vi "Task Manager.vi"() -> ()   [LabVIEW 2019, in "Task Manager.lvlib"]
doc: "This template is for the Queued Message Handler design pattern.\n\nThe Event Handling Loop generates messages based on user interface actions.\n\nThe Message Handling Loop processes messages generated by the Event Handling Loop, or by other messages. The messages are string values, so new messages can be added easily to the Message Cases case structure in the Message Handling Loop. Each message cluster can also provide an optional value for Message Data, which is a variant that can be converted to whatever message-specific data is required.a"
uses:
  Task Manager.lvlib
  Shared/TypeDefs/Queue Info.ctl
  Data.ctl
  Message Queue/State Name.ctl
  <vilib>/event_ctls.llb/usereventprio.ctl
  0c61461a-fa07-4497-8c8c-8d3ef654e9c8.vi
  bad579f2-958a-4e04-a1a5-1778729f7708.vi
  681f6a39-68c9-4eb8-ab39-fd2fc03f9966.vi
  <vilib>/Utility/error.llb/Clear Errors.vi
  Message Queue/Enqueue (Single).vi
  <vilib>/Utility/error.llb/Error Cluster From Error Code.vi
  Message Queue/Enqueue (Array).vi
  Message Queue/Reference Queue.vi
  Message Queue/Message Queue.lvlib
panel:
  in  "States Calling Info":cluster{"Queue Info":T1, "Show FP":bool}[](array[cluster])=[{"Queue Info"={"Module"="Asfand.lvlib", "State Name"="Initialize Data", "State Dequeue Time"="11 : 57 : 24.167319 AM", "Interval"="505.162129331m", "Call Chain"="Zeshan.lvlib:Zeshan.vi --> Message Queue.lvlib:Global Message Queue.vi", "# elements in queue"=0}, "Show FP"=FALSE}, {"Queue Info"={"Module"="Hamza.lvlib", "State Name"="[Event Structure] Update Data", "State Dequeue Time"="11 : 57 : 24.030312 AM", "Interval"="505.018426931m", "Call Chain"="Hamza.lvlib:Hamza.vi", "# elements in queue"=0}, "Show FP"=FALSE}, {"Queue Info"={"Module"="Zeshan.lvlib", "State Name"="[Event Structure] Update Data", "State Dequeue Time"="11 : 57 : 24.090315 AM", "Interval"="801.170772896m", "Call Chain"="Zeshan.lvlib:Zeshan.vi", "# elements in queue"=0}, "Show FP"=FALSE}]
  out "Modules Names":string[](array[string])=["Asfand", "Hamza", "Zeshan", "Acquire Mouse", "Task Manager"]
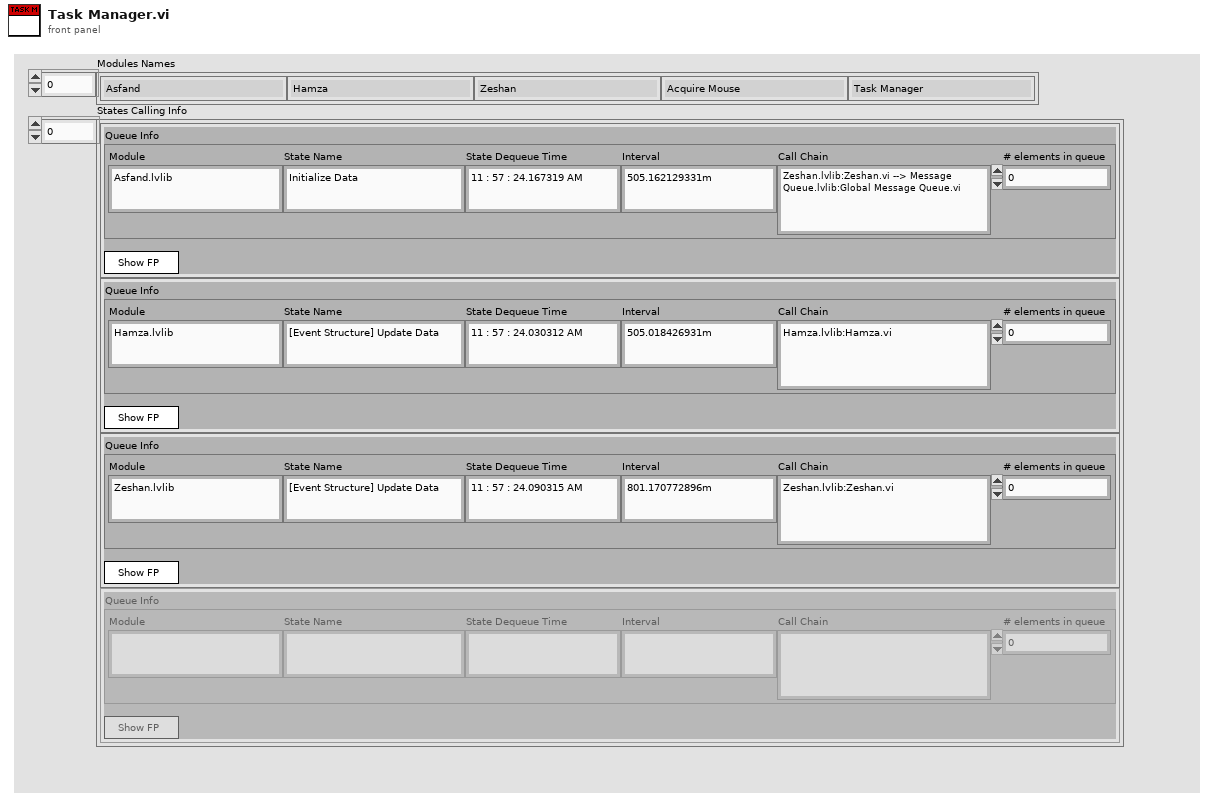
[diagram p1: front panel]
types:
  T1 = typedef "Queue Info.ctl" = cluster{"Module":string, "State Name":string, "State Dequeue Time":string, "Interval":string, "Call Chain":string, "# elements in queue":i32}
  T2 = typedef "Task Manager.lvlib/State Name.ctl" = enum16{"Default", "Initialize", "Re-Initialize", "Initialize Data", "Initialize Panel", "[Event Structure] Update Data", "Get Modules", "Add State Info Clone", "Get Queue Sizes", "Get States Calling Info", "Error", "Exit"}
  T3 = typedef "Task Manager.lvlib/Data.ctl" = cluster{"Exit":bool, "States":T2, "Refs":cluster{"Modules":refnum<vi>[], "FGVs":refnum<vi>[]}, "Modules":string[], "Queues Status":cluster{"max queue size":i32, "queue name":string, "# pending remove":i32, "# pending insert":i32, "# elements in queue":i32, "elements":cluster{"Custom State Name":string, "Defined State Name":variant, "Call Chain":string[], "Message Data":variant}[]}[], "States Calling Info":cluster{"Queue Info":T1, "Show FP":bool}[]}
  T4 = typedef "Message Queue Ref.ctl" = refnum<queue>
  T5 = typedef "Message Queue.lvlib/State Name.ctl" = enum16{"Default", "Initialize", "Initialize Data", "Initialize Modules", "Initialize Panel", "Close FP", "Open FP", "Initialize Menu", "Mode", "Update Subpanel", "Error", "Open Help", "About", "Open WebResources", "Exit"}
  T6 = typedef "usereventprio.ctl" = enum32{"high priority", "normal priority"}
  T7 = cluster{"max queue size":i32, "queue name":string, "# pending remove":i32, "# pending insert":i32, "# elements in queue":i32, "elements":cluster{"Custom State Name":string, "Defined State Name":variant, "Call Chain":string[], "Message Data":variant}[]}
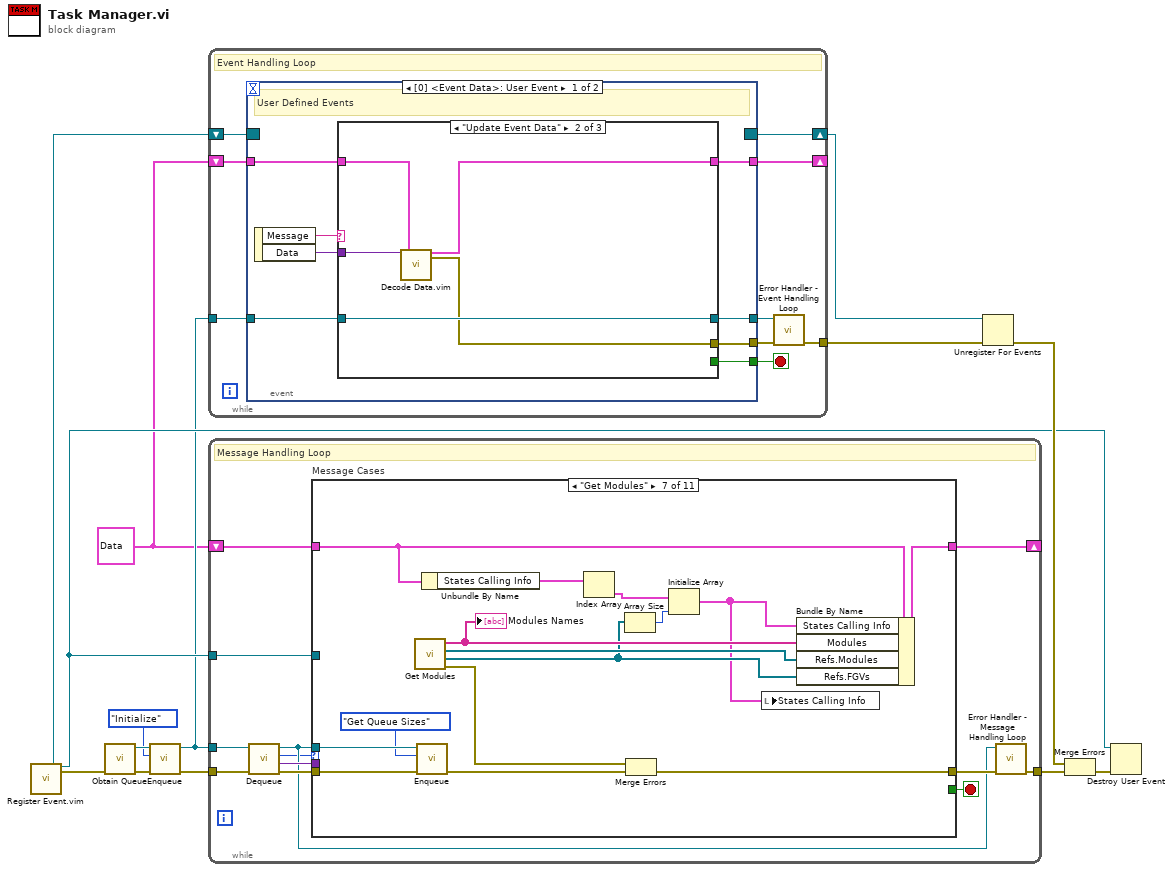
[diagram p0: block diagram]
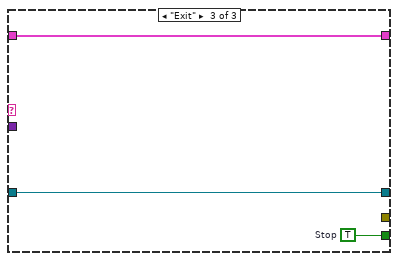
[diagram p3: hidden frame]
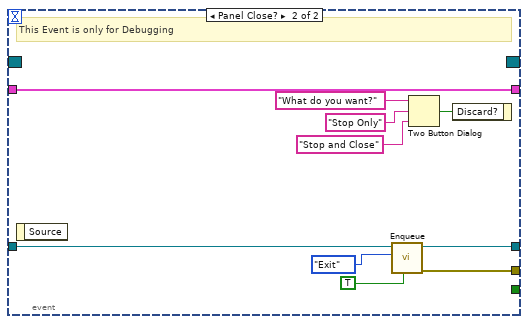
[diagram p4: hidden frame]
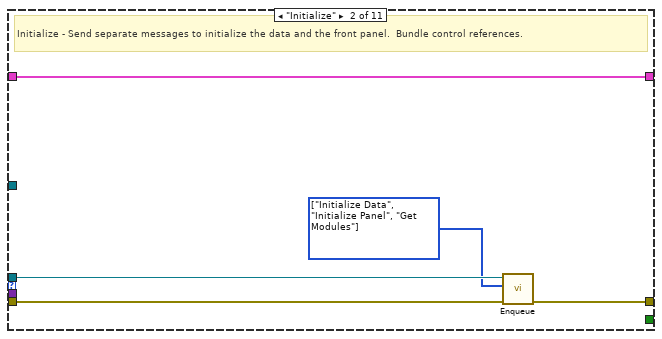
[diagram p6: hidden frame]
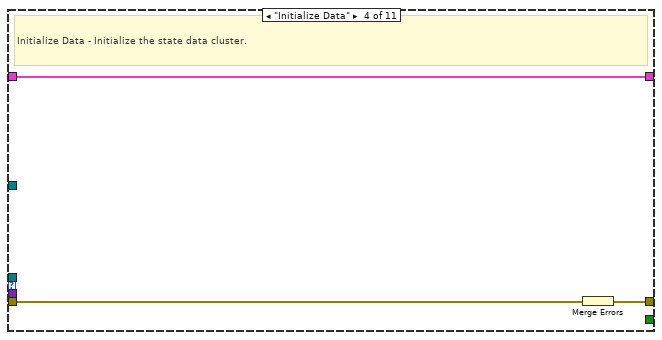
[diagram p8: hidden frame]
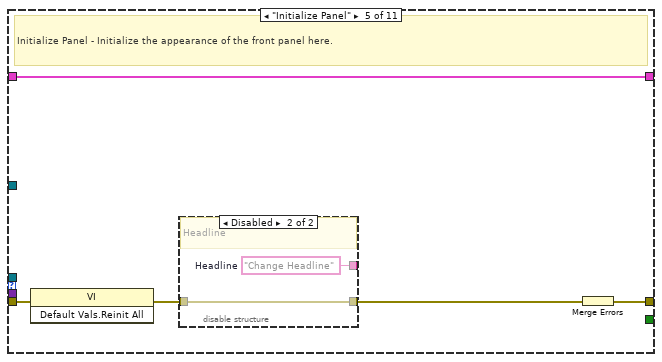
[diagram p9: hidden frame]
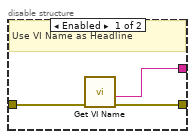
[diagram p10: hidden frame]
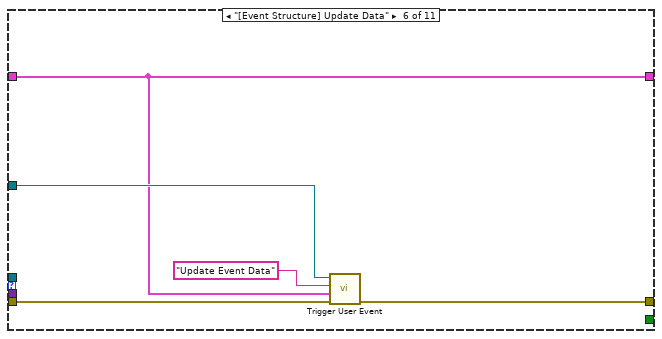
[diagram p11: hidden frame]
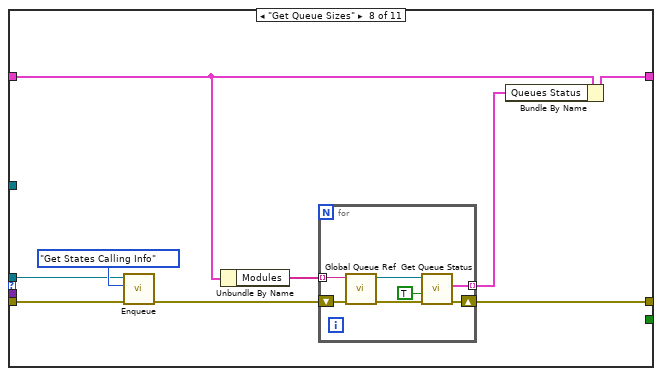
[diagram p12: hidden frame]
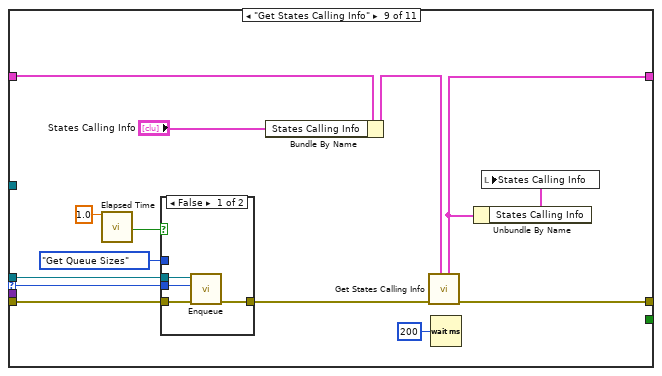
[diagram p13: hidden frame]
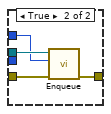
[diagram p14: hidden frame]
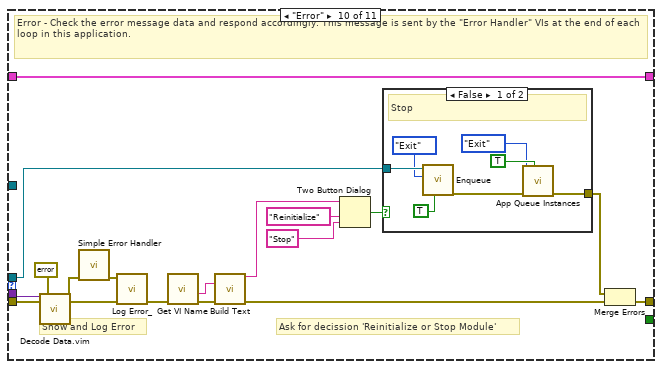
[diagram p15: hidden frame]
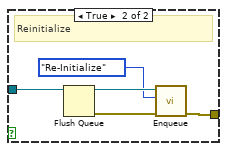
[diagram p16: hidden frame]
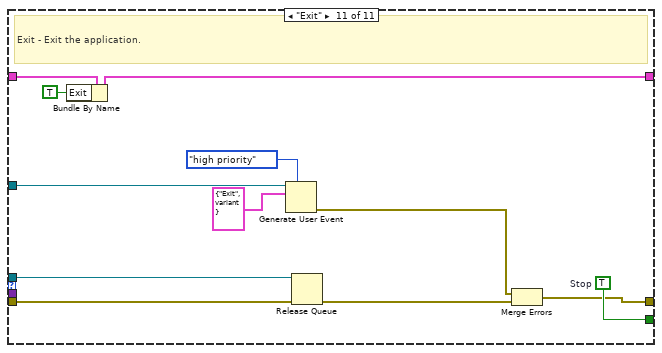
[diagram p17: hidden frame]
diagram:
  w3 = T3 {"Exit"=FALSE, "States"=enum."Initialize", "Refs"={"Modules"=[], "FGVs"=[]}, "Modules"=[], "Queues Status"=[], "States Calling Info"=[]} ("Data")
  n1 = call "Register Event.vim"() -> ("Registration"=w2:refnum<event-registration>, "user event out"=w5:refnum<user-event>, "error out"=w6:errorcluster)  [unwired: 17 in]
  n2 = call "Obtain Queue.vi"("error in (no error)"=w6) -> ("error out"=w10:errorcluster, "Message out"=w11:T4)  [unwired: 9 in]
  n3 = call-poly "Enqueue.vi"("error in (no error)"=w10, "States"=State_Name."Initialize", "Message Queue"=w11) -> ("error out"=w9:errorcluster, "Message Queue dub"=w4:T4)  [unwired: 7 in]
  n4 = while {
    tunnel: w4 -> [w23]
    shift-right: [w15] -> w8
    shift-left: w2 -> [w16]
    tunnel: [w20] -> w12
    shift-right: [w17] -> _
    shift-left: w3 -> [w18]
    stop <- w22 stop-if-true
    # "Event Handling Loop"
    n5 = event shown="[0] <Event Data>: User Event" {
      selector: w16 -> [_ _]
      dyn-events: [_ _] -> w15
      timeout: _ -> [_ _]
      tunnel: [w31 _] -> w22
      tunnel: w23 -> [w28 w44]
      tunnel: [w30 w45] -> w19
      tunnel: [w29 w46] -> w21
      tunnel: w18 -> [w26 w42]
      tunnel: [w27 w42] -> w17
      event User Event {
        # "User Defined Events"
        n6 = event-data() -> ("Message"=w25:string, "Data"=w24:variant)  [unwired: 1 in]
        n7 = case shown="\"Update Event Data\"" w25 {
          tunnel: [_ _ w41] -> w31
          tunnel: [_ w34 _] -> w30
          tunnel: w24 -> [_ w38 _]
          tunnel: [w33 w35 w40] -> w29
          tunnel: w28 -> [w33 w35 w40]
          tunnel: [w32 w36 w39] -> w27
          tunnel: w26 -> [w32 w37 w39]
          frame Default {
          }
          frame "Update Event Data" {
            n8 = call "Decode Data.vim"("Data"=w38, "Type/Default value"=w37) -> ("Data out"=w36:T3, "error out"=w34:errorcluster)  [unwired: 16 in]
          }
          frame "Exit" {
            w41 = TRUE  # Stop
          }
        }
      }
      event Panel Close? {
        # "This Event is only for Debugging"
        n9 = event-data() -> ()  [unwired: 1 in, 1 out]
        n10 = call-poly "Enqueue.vi"("Priority Message? Array"=TRUE ("Priority Message? (F)"), "States"=State_Name."Exit" ("Array"), "Message Queue"=w44) -> ("error out"=w45:errorcluster, "Message Queue dub"=w46:T4)  [unwired: 7 in]
        n11 = Two Button Dialog(message="What do you want?", 1:"Stop and Close" ("F button name (\"Cancel\")"), 2:"Stop Only" ("T button name (\"OK\")")) -> (T button?=w48:bool)
        n12 = event-data("Discard?"=w48) -> ()  [unwired: 1 in, 1 out]
      }
    }
    n13 = call "Error Handler - Event Handling Loop.vi"("error in (no error)"=w19, "Message Queue"=w21) -> ("dup error in"=w20:errorcluster)  [unwired: 8 in, 1 out]
  }
  n14 = while {
    tunnel: w4 -> [w58]
    tunnel: w9 -> [w61]
    tunnel: [w57] -> w14
    shift-right: [w53] -> _
    shift-left: w3 -> [w63]
    tunnel: w5 -> [w52]
    stop <- w62 stop-if-true
    # "Message Handling Loop"
    n15 = call "Dequeue.vi"("error in (no error)"=w61, "Message Queue"=w58) -> ("error out"=w60:errorcluster, "Message Data"=w59:variant, "State"=w54:T2, "Message Queue dub"=w55:T4)  [unwired: 4 in, 2 out]
    n16 = case "Message Cases" shown="\"Get Modules\"" w54 {
      selector: w54 -> [_ _ _ _ _ _ _ _ w128 _ _]
      tunnel: w55 -> [_ w68 _ _ _ _ w99 w106 w127 w150 w185]
      tunnel: w60 -> [w65 w69 w72 w73 w78 w90 w101 w109 w126 w148 w181]
      tunnel: [w65 w70 w72 w75 w80 w89 w103 w114 w135 w149 w182] -> w56
      tunnel: w63 -> [w64 w67 w71 w74 w79 w87 w97 w112 w134 w161 w179]
      tunnel: [_ _ _ _ _ _ _ _ _ _ w184] -> w62
      tunnel: w59 -> [_ _ _ _ _ _ _ _ _ w145 _]
      tunnel: [w64 w67 w71 w74 w79 w87 w105 w111 w133 w161 w175] -> w53
      tunnel: w52 -> [_ _ _ _ _ w88 _ _ _ _ w180]
      frame "Default", Default {
      }
      frame "Initialize" {
        w66 = T2[] [enum."Initialize Data", enum."Initialize Panel", enum."Get Modules"] items=["Default", "Initialize", "Re-Initialize", "Initialize Data", "Initialize Panel", "[Event Structure] Update Data", "Get Modules", "Add State Info Clone", "Get Queue Sizes", "Get States Calling Info", "Error", "Exit"] ("Array")
        # "Initialize - Send separate messages to initialize the data and the front panel.  Bundle control references."
        n17 = call-poly "Enqueue.vi"("error in (no error)"=w69, "States"=w66, "Message Queue"=w68) -> ("error out"=w70:errorcluster)  [unwired: 7 in, 1 out]
      }
      frame "Re-Initialize" {
      }
      frame "Initialize Data" {
        # "Initialize Data - Initialize the state data cluster."
        n18 = Merge Errors(w73) -> (w75:errorcluster)
      }
      frame "Initialize Panel" {
        # "Initialize Panel - Initialize the appearance of the front panel here."
        n19 = invoke class="VI" method="Default Vals.Reinit All"(error in=w78) -> (error out=w77:errorcluster)  [unwired: 2 in, 2 out]
        n20 = disable-structure shown="Disabled" {
          disable-tunnel: w77 -> [w83 w84]
          disable-tunnel: [w82 w84] -> w76
          disable-tunnel: [w81 w85] -> _
          frame Enabled {
            # "Use VI Name as Headline"
            n21 = call "Get VI Name.vi"("error in (no error)"=w83) -> ("error out"=w82:errorcluster, "VI Name without extension"=w81:string)  [unwired: 8 in, 1 out]
          }
          frame Disabled {
            w85 = "Change Headline"  # Headline
            # "Headline"
          }
        }
        n22 = Merge Errors(w76) -> (w80:errorcluster)
      }
      frame "[Event Structure] Update Data" {
        n23 = call "Trigger User Event.vi"("error in (no error)"=w90, "Message Data"=w87, "Message"="Update Event Data", "user event in"=w88) -> ("error out"=w89:errorcluster)  [unwired: 6 in, 1 out]
      }
      frame "Get Modules" {
        n24 = call "Get Modules.vi"() -> ("error out"=w102:errorcluster, "FGVs"=w92:refnum<vi>[], "Modules Refs"=w104:refnum<vi>[], "Modules Names"=w94:string[])  [unwired: 8 in]
        "Modules Names" <- w94
        n25 = call-poly "Enqueue.vi"("error in (no error)"=w101, "States"=State_Name."Get Queue Sizes", "Message Queue"=w99) -> ("error out"=w100:errorcluster)  [unwired: 7 in, 1 out]
        n26 = Unbundle By Name(w97) -> ("States Calling Info"=w96:cluster{"Queue Info":T1, "Show FP":bool}[])
        n27 = Index Array(array=w96) -> (element=w95:cluster{"Queue Info":T1, "Show FP":bool})  [unwired: 1 in]
        n28 = Array Size(array=w92) -> (size(s)=w93:i32)
        n29 = Merge Errors(w102, w100) -> (w103:errorcluster)
        n30 = Initialize Array(w95, w93) -> (w91:cluster{"Queue Info":T1, "Show FP":bool}[])
        n31 = local write "States Calling Info"(w91) -> ()
        n32 = Bundle By Name(cluster=w97, "States Calling Info"=w91, "Modules"=w94, "Refs.Modules"=w104, "Refs.FGVs"=w92) -> (w105:T3)
      }
      frame "Get Queue Sizes" {
        n33 = call-poly "Enqueue.vi"("error in (no error)"=w109, "States"=State_Name."Get States Calling Info", "Message Queue"=w106) -> ("error out"=w108:errorcluster)  [unwired: 7 in, 1 out]
        n34 = Unbundle By Name(w112) -> ("Modules"=w113:string[])
        n35 = for {
          shift-right: [w118] -> w114
          shift-left: w108 -> [w120]
          tunnel: w113 -> [w121] mode=indexing
          tunnel: [w115] -> w110 mode=indexing
          n36 = call "Global Queue Ref.vi"("error in (no error)"=w120, "Module Name"=w121) -> ("error out"=w119:errorcluster, "queue out"=w117:T4)  [unwired: 8 in]
          n37 = call "Get Queue Status.vi"("error in (no error)"=w119, "return elements? (T)"=TRUE, "Message Queue"=w117) -> ("error out"=w118:errorcluster, "Queue Status"=w115:T7)  [unwired: 6 in, 1 out]
        }
        n38 = Bundle By Name(cluster=w112, "Queues Status"=w110) -> (w111:T3)
      }
      frame "Get States Calling Info" {
        n39 = call "Elapsed Time"("Time Target (s)"=1.0) -> ("Time has Elapsed"=w129:bool)  [unwired: 11 in, 7 out]
        n40 = case shown="False" w129 {
          tunnel: w127 -> [w138 w143]
          tunnel: w126 -> [w137 w142]
          tunnel: [w136 w141] -> w132
          tunnel: State_Name."Get Queue Sizes" ("States") -> [_ w140]
          tunnel: w128 -> [w139 _]
          frame False {
            n41 = call-poly "Enqueue.vi"("error in (no error)"=w137, "States"=w139, "Message Queue"=w138) -> ("error out"=w136:errorcluster)  [unwired: 7 in, 1 out]
          }
          frame True {
            n42 = call-poly "Enqueue.vi"("error in (no error)"=w142, "States"=w140, "Message Queue"=w143) -> ("error out"=w141:errorcluster)  [unwired: 7 in, 1 out]
          }
        }
        n43 = Bundle By Name(cluster=w134, "States Calling Info"="States Calling Info") -> (w123:T3)
        n44 = call "Get States Calling Info.vi"("Data in"=w123, "error in (no error)"=w132) -> ("error out"=w135:errorcluster, "Data out"=w133:T3)  [unwired: 8 in]
        n45 = Wait (ms)(milliseconds to wait=u32 200) -> ()  [unwired: 1 out]
        n46 = Unbundle By Name(w133) -> ("States Calling Info"=w124:cluster{"Queue Info":T1, "Show FP":bool}[])
        n47 = local write "States Calling Info"(w124) -> ()
      }
      frame "Error" {
        # "Ask for decission 'Reinitialize or Stop Module'"
        # "Show and Log Error"
        # "Error - Check the error message data and respond accordingly. This message is sent by the \"Error Handler\" VIs at the end of each loop in this application."
        n48 = call "Decode Data.vim"("Data"=w145, "error in"=w148, "Type/Default value"=errorcluster {"status"=FALSE, "code"=0, "source"=""} ("error constant")) -> ("Data out"=w146:errorcluster, "error out"=w144:errorcluster)  [unwired: 15 in]
        n49 = call <vilib>:"Simple Error Handler.vi"("error in (no error)"=w146) -> ("error out"=w160:errorcluster)  [unwired: 4 in, 4 out]
        n50 = call "Log Error_.vi"("error in"=w144, "Error log to file"=w160) -> ("error out"=w159:errorcluster)  [unwired: 9 in]
        n51 = call "Get VI Name.vi"("error in (no error)"=w159) -> ("error out"=w155:errorcluster, "VI Name without extension"=w156:string)  [unwired: 8 in, 1 out]
        n52 = call "Build Text"("ModuleName"=w156, "error in (no error)"=w155) -> ("Result"=w158:string, "error out"=w157:errorcluster)  [unwired: 12 in]
        n53 = Two Button Dialog(message=w158, 1:"Stop" ("F button name (\"Cancel\")"), 2:"Reinitialize" ("T button name (\"OK\")")) -> (T button?=w154:bool)
        n54 = case shown="False" w154 {
          tunnel: w150 -> [w168 w173]
          tunnel: [w166 w170] -> w153
          frame False {
            # "Stop"
            n55 = call-poly "Enqueue.vi"("Priority Message? Array"=TRUE ("Priority Message? (F)"), "States"=State_Name."Exit" ("Array"), "Message Queue"=w168) -> ("error out"=w164:errorcluster)  [unwired: 7 in, 1 out]
            n56 = call-poly "App Queue Instances.vi"("Priority Message? (F)"=TRUE, "error in (no error)"=w164, "Tasks"=State_Name."Exit") -> ("error out"=w166:errorcluster)  [unwired: 8 in]
          }
          frame True {
            # "Reinitialize"
            n57 = Flush Queue(queue=w173) -> (queue out=w172:T4, error out=w171:errorcluster)  [unwired: 1 in, 1 out]
            n58 = call-poly "Enqueue.vi"("error in (no error)"=w171, "States"=State_Name."Re-Initialize" ("Array"), "Message Queue"=w172) -> ("error out"=w170:errorcluster)  [unwired: 7 in, 1 out]
          }
        }
        n59 = Merge Errors(w153, w157) -> (w149:errorcluster)
      }
      frame "Exit" {
        w184 = TRUE  # Stop
        # "Exit - Exit the application."
        n60 = Bundle By Name(cluster=w179, "Exit"=TRUE) -> (w175:T3)
        n61 = Generate User Event(priority (normal)=usereventprio."high priority", user event=w180, event data cluster=cluster{"Message":string, "Data":variant} {"Message"="Exit", "Data"=variant} ("event data")) -> (error out=w177:errorcluster)  [unwired: 1 in, 1 out]
        n62 = Release Queue(queue=w185, error in (no error)=w181) -> (error out=w183:errorcluster)  [unwired: 1 in, 2 out]
        n63 = Merge Errors(w177, w183) -> (w182:errorcluster)
      }
    }
    n64 = call "Error Handler - Message Handling Loop.vi"("error in (no error)"=w56, "Message Queue"=w55) -> ("dup error in"=w57:errorcluster)  [unwired: 8 in, 1 out]
  }
  n65 = Unregister For Events(event registration refnum=w8, error in=w12) -> (error out=w13:errorcluster)
  n66 = Merge Errors(w13, w14) -> (w7:errorcluster)
  n67 = Destroy User Event(user event=w5, error in=w7) -> ()  [unwired: 1 out]
